vi "To Default.vi"(8 "error in (no error)":errorcluster, 11 "Request Data in":refnum<class "Request Data.lvclass">) -> (0 "error dub":errorcluster, 3 "Request Data out":refnum<class "Request Data.lvclass">)   [LabVIEW 2020, in "Publisher.lvlib" / "Request Data.lvclass"]
doc: "Restore class data to the default value."
uses:
  Request Data.lvclass
  Request Data.lvclass/Request Data.ctl
  PPL/HDH.Data.Generic.lvlibp/Data.lvclass
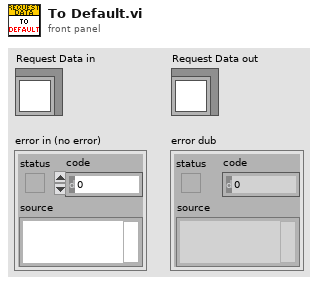
[diagram p1: front panel]
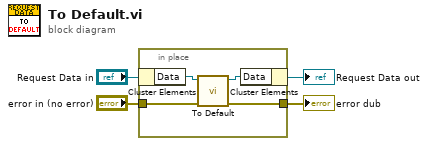
[diagram p0: block diagram]
diagram:
  n1 = in-place {
    in-place-border: "error in (no error)" -> [w6]
    in-place-border: [w5] -> w1
    n2 = in-place-cluster #1("Request Data in") -> ("Data"=w8:refnum<class "Data.lvclass">)
    n3 = call-dynamic "To Default.vi"("error in (no error)"=w6, "Data in"=w8) -> ("error dub"=w5:errorcluster, "Data out"=w7:refnum<class "Data.lvclass">)  [unwired: 8 in]
    n4 = in-place-cluster #1("Data"=w7) -> (→"Request Data out":refnum<class "Request Data.lvclass">)
  }
  "error dub" <- w1
